vi "Read from COM Port.vi"(8 "error in":errorcluster caption="error IO", 10 "Byte to Read (-1:All)":i32, 11 "VISA resource name in":refnum<visa-resource-name>) -> (0 "error out":errorcluster, 1 "readed Bytes":u32, 2 "String (output)":string, 3 "VISA resource name out":refnum<visa-resource-name>)   [LabVIEW 2015, in "JULABO DeviceDriver.lvlib"]
uses:
  JULABO DeviceDriver.lvlib
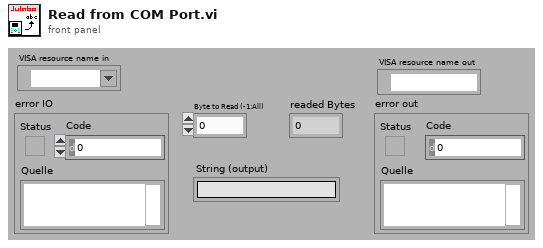
[diagram p1: front panel]
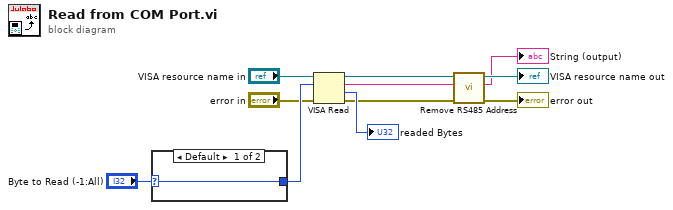
[diagram p0: block diagram]
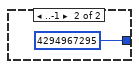
[diagram p2: hidden frame]
diagram:
  n1 = case shown="Default" "Byte to Read (-1:All)" {
    selector: "Byte to Read (-1:All)" -> [w12 _]
    tunnel: [w12 u32 4294967295 ("Anzahl der Bytes")] -> w9
    frame Default {
    }
    frame ..-1 {
    }
  }
  n2 = VISA Read(VISA resource name="VISA resource name in", byte count=w9, error in (no error)="error in") -> (VISA resource name out=w6:refnum<visa-resource-name>, read buffer=w1:string, return count=→"readed Bytes":u32, error out=w5:errorcluster)
  n3 = call "Remove RS485 Address.vi"("error in"=w5, "Command (input)"=w1, "VISA resource name in"=w6) -> ("error out"=→"error out":errorcluster, "Command (output)"=→"String (output)":string, "VISA resource name out"=→"VISA resource name out":refnum<visa-resource-name>)  [unwired: 2 in]
